vi "Init_Control.vi"(8 "error in (no error)":errorcluster) -> (0 "error out":errorcluster, 1 "App.SaveVersions":string[](array[string]), 2 "Styles strings":string[](array[string]), 3 "Control out":refnum<class "Control.lvclass">)   [LabVIEW 2013, in "uitools_Control.lvlib" / "Control.lvclass"]
uses:
  Control.lvclass
  Typedefs/TypeDef_Action.ctl
  <userlib>/BitMan/BitMap class/BitMap.lvclass
  Controls/_ui_tools_font.ctl
  Controls/BX.Orientation__LCR _Modified.ctl
  Control.lvclass/Control.ctl
  <userlib>/_OpenG.lib/array/array.llb/Conditional Auto-Indexing Tunnel (String)__ogtk.vi
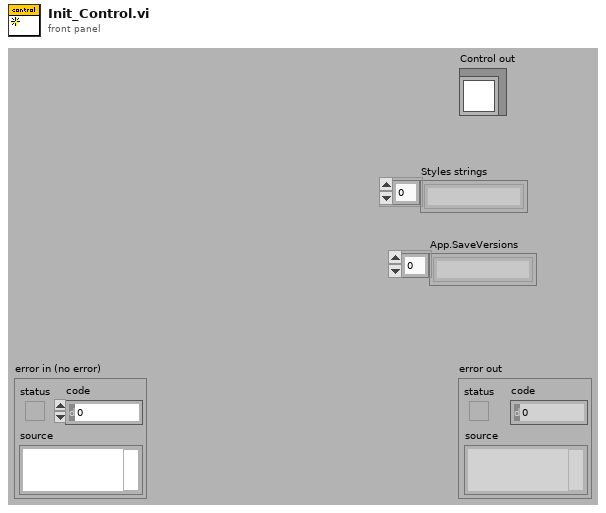
[diagram p1: front panel]
types:
  T1 = typedef "uitools_Control.lvlib/Control.lvclass/BX.Orientation__LCR _Modified.ctl" = u8
  T2 = typedef "uitools_Control.lvlib/Control.lvclass/_ui_tools_font.ctl" = cluster{"Font Name:":string, "Size":i16, "Strikeout?":bool, "Italic?":bool, "Underline?":bool, "Outline?":bool, "Shadow?":bool, "Bold?":bool}
  T3 = typedef "uitools_Control.lvlib/Control.lvclass/TypeDef_Action.ctl" = u16
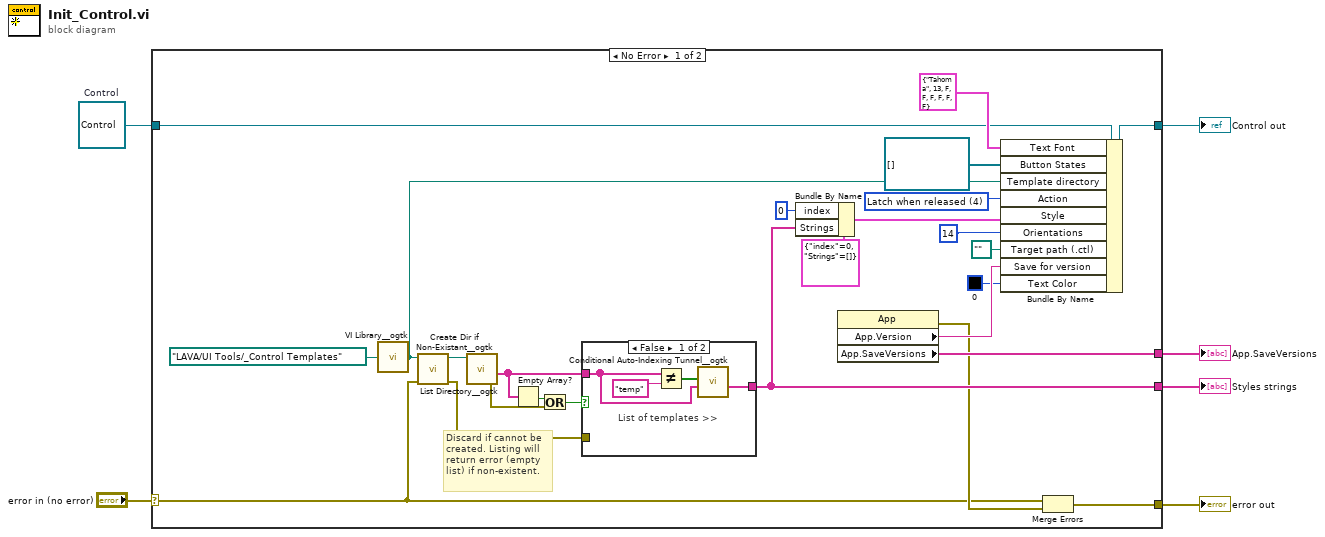
[diagram p0: block diagram]
diagram:
  w2 = refnum<class "Control.lvclass"> refnum  # Control
  n1 = case shown="No Error" "error in (no error)" {
    selector: "error in (no error)" -> [w14 w37]
    tunnel: [w13 w37] -> w6
    tunnel: [w7 w36] -> w5
    tunnel: w2 -> [w25 w36]
    tunnel: [w24 _] -> w4
    tunnel: [w20 _] -> w1
    frame No Error {
      w21 = T3 4 items=["Switch when pressed", "Switch when released", "Switch until release", "Latch when pressed", "Latch when released", "Latch until released"] ("Action")
      # "Discard if cannot be\ncreated. Listing will\nreturn error (empty\nlist) if non-existent."
      n2 = call <userlib>:"VI Library__ogtk.vi"("Relative path (.)"=path "LAVA/UI Tools/_Control Templates") -> ("VI Library (+ Relative)"=w16:path)
      n3 = call <userlib>:"Create Dir if Non-Existant__ogtk.vi"("error in (no error)"=w14, "Directory Path"=w16) -> ("error out"=w8:errorcluster, "dup Directory Path"=w22:path)  [unwired: 1 in, 7 out]
      n4 = call <userlib>:"List Directory__ogtk.vi"("directory path"=w22) -> ("error out"=w9:errorcluster, "directory names"=w10:string[])  [unwired: 2 in, 3 out]
      n5 = Empty Array?(array=w10) -> (empty?=w11:bool)
      n6 = Or(x=w11, y=w9) -> (x .or. y?=w12:bool)
      n7 = case shown="False" w12 {
        tunnel: w10 -> [w33 _]
        tunnel: [w32 _] -> w24
        tunnel: w8 -> [_ _]
        frame False {
          # "List of templates >>"
          n8 = Not Equal?(x=w33, y="temp") -> (x != y?=w34:bool[])
          n9 = call-poly <userlib>:"Conditional Auto-Indexing Tunnel__ogtk.vi"("Array in"=w33, "Elements to keep"=w34) -> ("Filtered Array out"=w32:string[])  [unwired: 5 out]
        }
        frame True {
          # "Empty\nNo templates found."
        }
      }
      n10 = Bundle By Name(cluster=cluster{"index":u16, "Strings":string[]} {"index"=0, "Strings"=[]} ("Style"), "index"=u16 0, "Strings"=w24) -> (w31:cluster{"index":u16, "Strings":string[]})
      n11 = property class="App"() -> (error out=w15:errorcluster, "App.Version"=w19:string, "App.SaveVersions"=w20:string[])  [unwired: 2 in, 1 out]
      n12 = Bundle By Name(cluster=w25, "Text Font"=T2 {"Font Name:"="Tahoma", "Size"=13, "Strikeout?"=FALSE, "Italic?"=FALSE, "Underline?"=FALSE, "Outline?"=FALSE, "Shadow?"=FALSE, "Bold?"=FALSE} ("Font"), "Button States"=refnum<class "BitMap.lvclass">[] [], "Template directory"=w16, "Action"=w21, "Style"=w31, "Orientations"=T1 14, "Target path (.ctl)"=path "", "Save for version"=w19, "Text Color"=u32 0) -> (w7:refnum<class "Control.lvclass">)
      n13 = Merge Errors(w14, w15) -> (w13:errorcluster)
    }
    frame Error {
    }
  }
  "error out" <- w6
  "Control out" <- w5
  "Styles strings" <- w4
  "App.SaveVersions" <- w1
